vi "Path format.vi"(2 "Operation type":u8(ring) items=["Equalization", "Acquisition"], 3 "HV level":i16, 4 "I leakage":u8 max=3, 5 "HV enable button":bool caption="High Voltage enable") -> (0 "folder path":path)   [LabVIEW 2015, in "VIPM2.lvlib"]
doc: "Build the folder path.\nC:\\VIP Module\\Files\\Equalization\\yyyymmdd_hh-mm-ss_Leak#_HV#\\\nC:\\VIP Module\\Files\\Acquisition\\yyyymmdd_hh-mm-ss_Leak#_HV#\\\nCreate path if it doesn't exist."
uses:
  VIPM2.lvlib
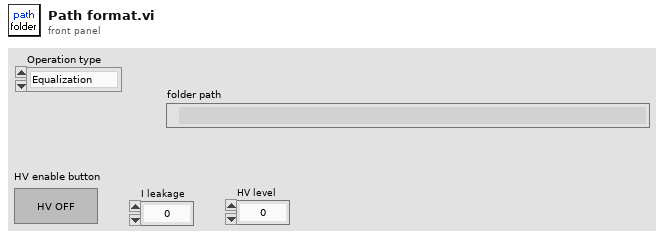
[diagram p1: front panel]
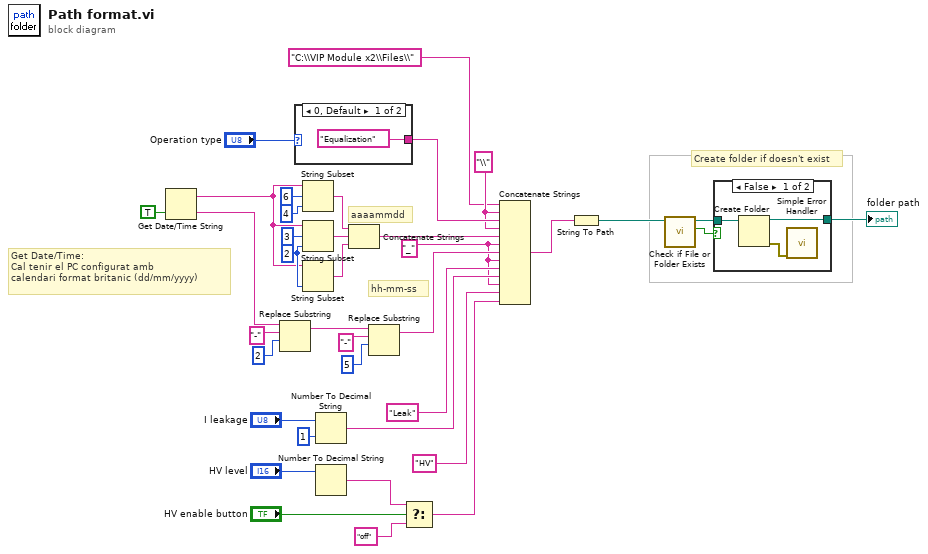
[diagram p0: block diagram]
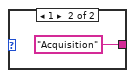
[diagram p3: hidden frame]
diagram:
  w8 = "_" ("string")
  w16 = "\\" ("string")
  w30 = 2 ("length (rest)")
  # "Create folder if doesn't exist"
  # "Get Date/Time:\nCal tenir el PC configurat amb\ncalendari format britanic (dd/mm/yyyy)"
  # "hh-mm-ss"
  # "aaaammdd"
  n1 = Get Date/Time String(want seconds? (F)=TRUE) -> (date string=w29:string, time string=w34:string)  [unwired: 2 in]
  n2 = Replace Substring(3:2 ("offset (0)"), 4:"-" ("substring (\"\")"), 5:w34) -> (1:w22:string)  [unwired: 1 in, 1 out]
  n3 = case shown="0, Default" "Operation type" {
    tunnel: ["Equalization" ("string") "Acquisition" ("string")] -> w24
    frame 0, Default {
    }
    frame 1 {
    }
  }
  n4 = String Subset(string=w29, offset (0)=6, length (rest)=4 ("length (rest)")) -> (substring=w31:string)
  n5 = String Subset(string=w29, offset (0)=3, length (rest)=w30) -> (substring=w32:string)
  n6 = String Subset(string=w29, length (rest)=w30) -> (substring=w33:string)  [unwired: 1 in]
  n7 = Number To Decimal String(number="I leakage", width (-)=i16 1) -> (decimal integer string=w9:string)
  n8 = Number To Decimal String(number="HV level") -> (decimal integer string=w4:string)  [unwired: 1 in]
  n9 = Concatenate Strings(w31, w32, w33) -> (w37:string)
  n10 = Replace Substring(3:5 ("offset (0)"), 4:"-" ("substring (\"\")"), 5:w22) -> (1:w21:string)  [unwired: 1 in, 1 out]
  n11 = Select(t=w4, s="HV enable button", f="off") -> (s? t:f=w2:string)
  n12 = Concatenate Strings "Concatenate Strings"("C:\\VIP Module x2\\Files\\" ("string"), w16, w24, w16, w37, w8, w21, w8, "Leak" ("string"), w9, w8, "HV" ("string"), w2) -> (w15:string)
  n13 = String To Path(string=w15) -> (path=w14:path)
  n14 = call <vilib>:"Check if File or Folder Exists.vi"("path"=w14) -> ("file or folder exists?"=w17:bool, "dup path"=w18:path)  [unwired: 8 in, 1 out]
  n15 = case shown="False" w17 {
    tunnel: w18 -> [w42 w43]
    tunnel: [w41 w43] -> w13
    frame False {
      n16 = Create Folder(path (use dialog)=w42) -> (created path=w41:path, error out=w40:errorcluster)  [unwired: 2 in, 1 out]
      n17 = call <vilib>:"Simple Error Handler.vi"("error in (no error)"=w40) -> ()  [unwired: 4 in, 5 out]
    }
    frame True {
    }
  }
  "folder path" <- w13
